vi "CreateUserEvents.vi"(1 "EventsReference in":T1) -> (0 "EventsReference out":T1)   [LabVIEW 2017, in "ImageAcquisitionLibrary.lvlib"]
uses:
  ImageAcquisitionProgram/ImageAcquisitionLibrary/ImageAcquisitionLibrary.lvlib
  EventsReference.ctl
  InterfaceReferences.ctl
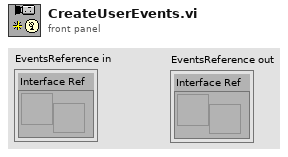
[diagram p1: front panel]
types:
  T1 = typedef "ImageAcquisitionLibrary.lvlib/EventsReference.ctl" = cluster{"Interface Ref":refnum<user-event>}
  T2 = typedef "ImageAcquisitionLibrary.lvlib/InterfaceReferences.ctl" = cluster{"Settings":refnum<vi>, "Acquire":refnum<vi>, "Record":refnum<vi>, "ImDisplay":refnum<vi>, "Messages":refnum<vi>, "Stop":refnum<vi>, "Tracking":refnum<vi>}
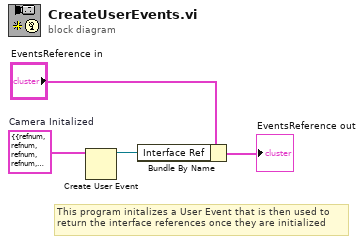
[diagram p0: block diagram]
diagram:
  w2 = cluster{"Camera Controls":T2} {"Camera Controls"={"Settings"=refnum, "Acquire"=refnum, "Record"=refnum, "ImDisplay"=refnum, "Messages"=refnum, "Stop"=refnum, "Tracking"=refnum}}  # Camera Initalized
  # "This program initalizes a User Event that is then used to\nreturn the interface references once they are initialized"
  n1 = Create User Event(user event datatype=w2) -> (user event=w1:refnum<user-event>)  [unwired: 1 in, 1 out]
  n2 = Bundle By Name(cluster="EventsReference in", "Interface Ref"=w1) -> (→"EventsReference out":T1)
